vi "A33ConfigureFSweep.vi"(0 "VISA resource name":refnum<visa-resource-name>="USB0::0x0957::0x5707::MY53800847::INSTR", 1 "Enable Frequency Sweep (T:Enable)":bool=TRUE, 2 "Sweep Time (1.0 Seconds)":dbl=1.0 format="%#.6g", 5 "Channel (1: Channel1)":u16(ring)=1 items=["Channel1"=1, "Channel2"=2], 7 "Sweep Spacing (0: Linear)":u16(ring) items=["Linear", "Logarithmic"], 9 "Start Frequency (1.0 uHz)":dbl=1e-06 format="%#.12g", 11 "error in (no error)":errorcluster, 12 "Stop  Frequency  (1000.0 Hz)":dbl=1000.0 format="%#.12g", 13 "Hold Time (0 Seconds)":dbl format="%#.6g", 14 "Return Time (0 Seconds)":dbl format="%#.6g") -> (4 "VISA resource name out":refnum<visa-resource-name>, 15 "error out":errorcluster)   [LabVIEW 2022 SP3]
doc: "Configures and enables a frequency sweep. In the frequency sweep mode, the function generator steps from the start frequency to the stop frequency at a sweep rate."
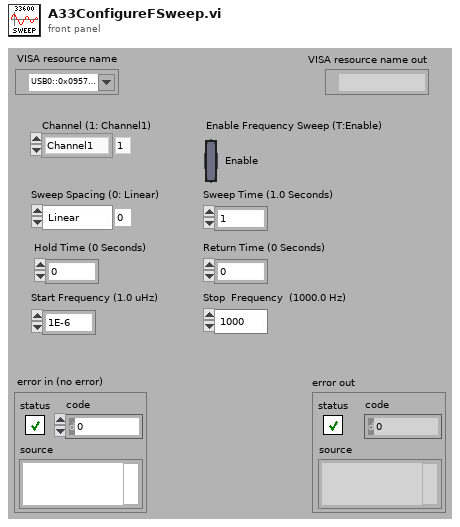
[diagram p1: front panel]
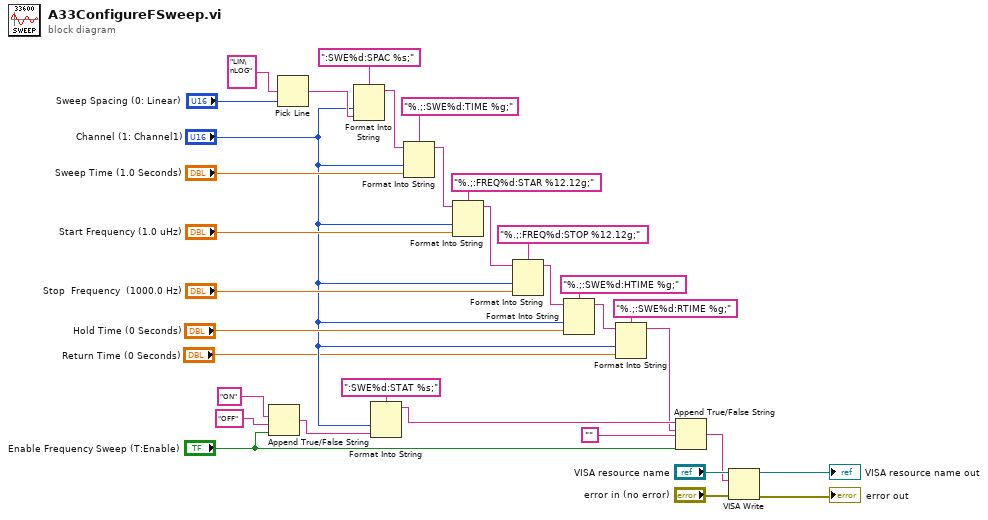
[diagram p0: block diagram]
diagram:
  n1 = Append True/False String(1:"Enable Frequency Sweep (T:Enable)", 2:"OFF", 3:"ON") -> (0:w13:string)  [unwired: 1 in]
  n2 = Pick Line(multi-line string="LIN\nLOG", line index="Sweep Spacing (0: Linear)") -> (output string=w30:string)  [unwired: 1 in]
  n3 = Format Into String(format string=":SWE%d:SPAC %s;", "Channel (1: Channel1)", w30) -> (resulting string=w27:string)  [unwired: 2 in, 1 out]
  n4 = Format Into String(format string=":SWE%d:STAT %s;", "Channel (1: Channel1)", w13) -> (resulting string=w17:string)  [unwired: 2 in, 1 out]
  n5 = Format Into String(format string="%.;:SWE%d:TIME %g;", initial string=w27, "Channel (1: Channel1)", "Sweep Time (1.0 Seconds)") -> (resulting string=w21:string)  [unwired: 1 in, 1 out]
  n6 = Format Into String(format string="%.;:FREQ%d:STAR %12.12g;", initial string=w21, "Channel (1: Channel1)", "Start Frequency (1.0 uHz)") -> (resulting string=w24:string)  [unwired: 1 in, 1 out]
  n7 = Format Into String(format string="%.;:FREQ%d:STOP %12.12g;", initial string=w24, "Channel (1: Channel1)", "Stop  Frequency  (1000.0 Hz)") -> (resulting string=w8:string)  [unwired: 1 in, 1 out]
  n8 = Format Into String(format string="%.;:SWE%d:HTIME %g;", initial string=w8, "Channel (1: Channel1)", "Hold Time (0 Seconds)") -> (resulting string=w4:string)  [unwired: 1 in, 1 out]
  n9 = Format Into String(format string="%.;:SWE%d:RTIME %g;", initial string=w4, "Channel (1: Channel1)", "Return Time (0 Seconds)") -> (resulting string=w1:string)  [unwired: 1 in, 1 out]
  n10 = Append True/False String(1:"Enable Frequency Sweep (T:Enable)", 2:"", 3:w1, 4:w17) -> (0:w16:string)
  n11 = VISA Write(VISA resource name="VISA resource name", write buffer=w16, error in (no error)="error in (no error)") -> (VISA resource name out=→"VISA resource name out":refnum<visa-resource-name>, error out=→"error out":errorcluster)  [unwired: 1 out]
